vi "StudentCode.vi"(0 "Sensor 1 Mode":dbl, 1 "Sensor 1 Value":dbl, 2 "Sensor 2 Mode":dbl, 3 "Sensor 2 Value":dbl) -> (15 "Motor 1 Value":dbl, 16 "Motor On Duration":dbl, 18 "Motor 2 Value":dbl)   [LabVIEW 2016]
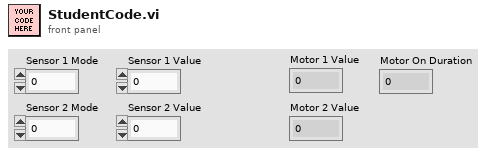
[diagram p1: front panel]
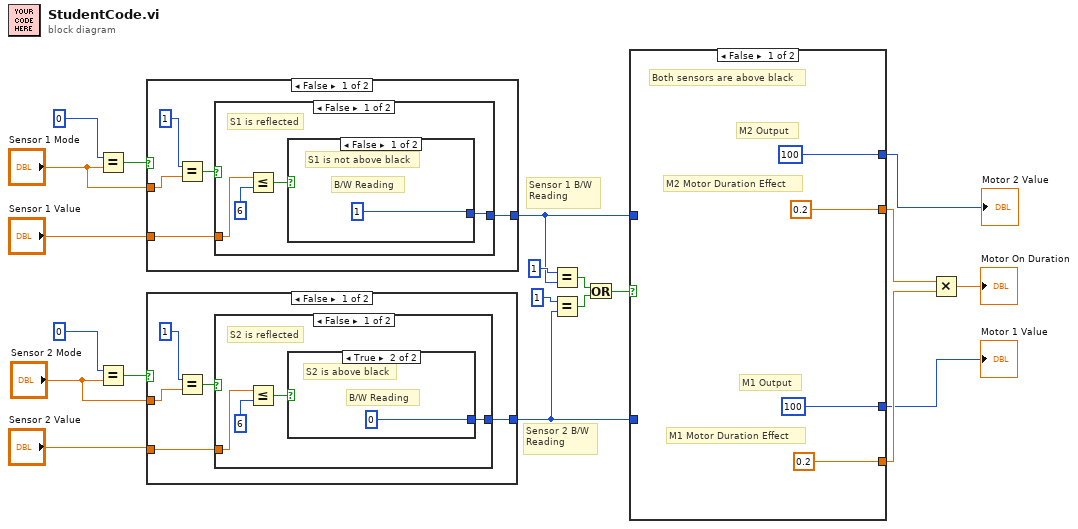
[diagram p0: block diagram]
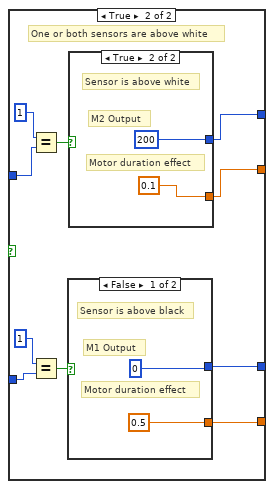
[diagram p2: hidden frame]
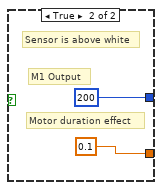
[diagram p3: hidden frame]
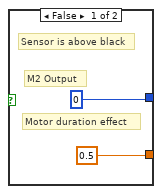
[diagram p4: hidden frame]
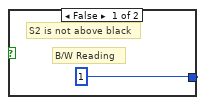
[diagram p5: hidden frame]
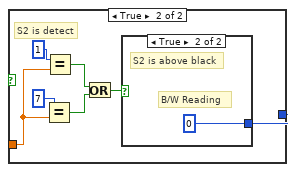
[diagram p6: hidden frame]
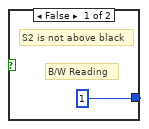
[diagram p7: hidden frame]
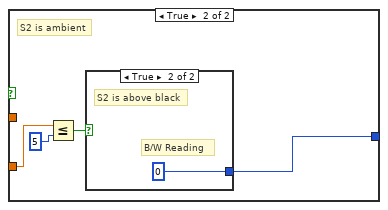
[diagram p8: hidden frame]
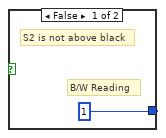
[diagram p9: hidden frame]
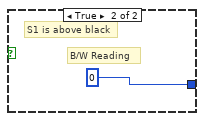
[diagram p10: hidden frame]
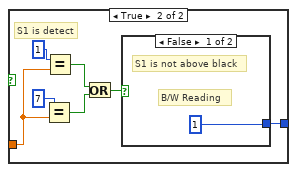
[diagram p11: hidden frame]
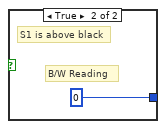
[diagram p12: hidden frame]
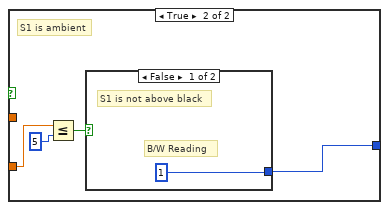
[diagram p13: hidden frame]
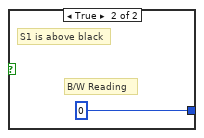
[diagram p14: hidden frame]
diagram:
  # "Sensor 2 B/W\nReading"
  # "Sensor 1 B/W\nReading"
  n1 = Equal?(x=0, y="Sensor 1 Mode") -> (x = y?=w19:bool)
  n2 = Equal?(x=0, y="Sensor 2 Mode") -> (x = y?=w15:bool)
  n3 = case shown="False" w19 {
    tunnel: "Sensor 1 Value" -> [w22 w44]
    tunnel: [w21 w41] -> w2
    tunnel: "Sensor 1 Mode" -> [w24 _]
    frame False {
      n4 = Equal?(x=1, y=w24) -> (x = y?=w23:bool)
      n5 = case shown="False" w23 {
        tunnel: w22 -> [w28 w36]
        tunnel: [w26 w32] -> w21
        frame False {
          # "S1 is reflected"
          n6 = Less Or Equal?(x=w28, y=6) -> (x <= y?=w27:bool)
          n7 = case shown="False" w27 {
            tunnel: [1 0] -> w26
            frame False {
              # "B/W Reading"
              # "S1 is not above black"
            }
            frame True {
              # "B/W Reading"
              # "S1 is above black"
            }
          }
        }
        frame True {
          # "S1 is detect"
          n8 = Equal?(x=7, y=w36) -> (x = y?=w37:bool)
          n9 = Equal?(x=1, y=w36) -> (x = y?=w38:bool)
          n10 = Or(x=w38, y=w37) -> (x .or. y?=w33:bool)
          n11 = case shown="False" w33 {
            tunnel: [1 0] -> w32
            frame False {
              # "B/W Reading"
              # "S1 is not above black"
            }
            frame True {
              # "B/W Reading"
              # "S1 is above black"
            }
          }
        }
      }
    }
    frame True {
      # "S1 is ambient"
      n12 = Less Or Equal?(x=w44, y=5) -> (x <= y?=w42:bool)
      n13 = case shown="False" w42 {
        tunnel: [1 0] -> w41
        frame False {
          # "B/W Reading"
          # "S1 is not above black"
        }
        frame True {
          # "B/W Reading"
          # "S1 is above black"
        }
      }
    }
  }
  n14 = case shown="False" w15 {
    tunnel: "Sensor 2 Value" -> [w48 w70]
    tunnel: [w47 w67] -> w1
    tunnel: "Sensor 2 Mode" -> [w50 _]
    frame False {
      n15 = Equal?(x=1, y=w50) -> (x = y?=w49:bool)
      n16 = case shown="False" w49 {
        tunnel: w48 -> [w54 w62]
        tunnel: [w52 w58] -> w47
        frame False {
          # "S2 is reflected"
          n17 = Less Or Equal?(x=w54, y=6) -> (x <= y?=w53:bool)
          n18 = case shown="True" w53 {
            tunnel: [1 0] -> w52
            frame False {
              # "B/W Reading"
              # "S2 is not above black"
            }
            frame True {
              # "B/W Reading"
              # "S2 is above black"
            }
          }
        }
        frame True {
          # "S2 is detect"
          n19 = Equal?(x=7, y=w62) -> (x = y?=w63:bool)
          n20 = Equal?(x=1, y=w62) -> (x = y?=w64:bool)
          n21 = Or(x=w64, y=w63) -> (x .or. y?=w59:bool)
          n22 = case shown="True" w59 {
            tunnel: [1 0] -> w58
            frame False {
              # "B/W Reading"
              # "S2 is not above black"
            }
            frame True {
              # "B/W Reading"
              # "S2 is above black"
            }
          }
        }
      }
    }
    frame True {
      # "S2 is ambient"
      n23 = Less Or Equal?(x=w70, y=5) -> (x <= y?=w68:bool)
      n24 = case shown="True" w68 {
        tunnel: [1 0] -> w67
        frame False {
          # "B/W Reading"
          # "S2 is not above black"
        }
        frame True {
          # "B/W Reading"
          # "S2 is above black"
        }
      }
    }
  }
  n25 = Equal?(x=1, y=w2) -> (x = y?=w9:bool)
  n26 = Equal?(x=1, y=w1) -> (x = y?=w8:bool)
  n27 = Or(x=w9, y=w8) -> (x .or. y?=w7:bool)
  n28 = case shown="False" w7 {
    tunnel: [100 w86] -> w3
    tunnel: [0.2 w85] -> w6
    tunnel: [100 w84] -> w4
    tunnel: [0.2 w83] -> w5
    tunnel: w2 -> [_ w81]
    tunnel: w1 -> [_ w78]
    frame False {
      # "M1 Motor Duration Effect"
      # "M1 Output"
      # "M2 Motor Duration Effect"
      # "M2 Output"
      # "Both sensors are above black"
    }
    frame True {
      # "One or both sensors are above white"
      n29 = Equal?(x=1, y=w81) -> (x = y?=w80:bool)
      n30 = Equal?(x=1, y=w78) -> (x = y?=w77:bool)
      n31 = case shown="False" w77 {
        tunnel: [0 200] -> w84
        tunnel: [0.5 0.1] -> w83
        frame False {
          # "Motor duration effect"
          # "M1 Output"
          # "Sensor is above black"
        }
        frame True {
          # "Motor duration effect"
          # "M1 Output"
          # "Sensor is above white"
        }
      }
      n32 = case shown="True" w80 {
        tunnel: [0 200] -> w86
        tunnel: [0.5 0.1] -> w85
        frame False {
          # "Motor duration effect"
          # "M2 Output"
          # "Sensor is above black"
        }
        frame True {
          # "Motor duration effect"
          # "M2 Output"
          # "Sensor is above white"
        }
      }
    }
  }
  "Motor 1 Value" <- w4
  "Motor 2 Value" <- w3
  n33 = Multiply(x=w6, y=w5) -> (x*y=→"Motor On Duration":dbl)
